vi "PixyGetCube.vi"(10 "AbortButtonPushed":bool, 11 "CubeGrabButtonPushed":bool) -> (3 "GotCube?":bool)   [LabVIEW 2017]
uses:
  <vilib>/Rock Robotics/SystemInterfaces/i2clib/i2c_bus.ctl
panel:
  in  "EndCondArea":i32=11000
  in  "CenterSetpoint":i32=80
  in  "AreaSetpoint":i32
  in  "MaxY":i32=130
  in  "KdX":dbl=0.07
  in  "MaxSpeed":dbl=0.3
  in  "KpX":dbl=0.1
  in  "KpY":dbl=0.0001
  in  "Pixy Address":u8=84 format="%x"
  # "320 x 200"
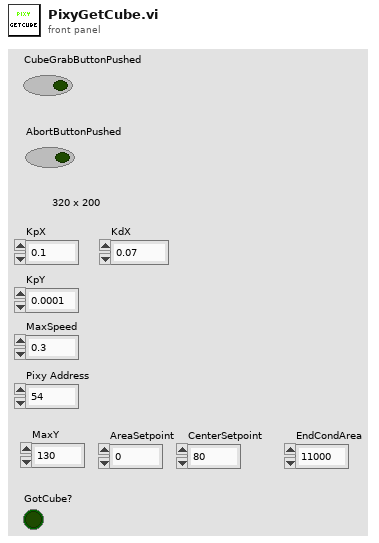
[diagram p1: front panel]
types:
  T1 = typedef "i2c_bus.ctl" = enum16{"I2C On-Board", "I2C MXP", "Invalid"}
  T2 = typedef "WPI_MotorControlDeviceRef.ctl" = cluster{"DeviceStatus":errorcluster, "Type":T3, "PWM":cluster{"PWM Channel":T4, "DeadBand":T5}, "CAN":cluster{"Device Number":u8, "SetOutput VI Ref":variant, "GetOutput VI Ref":variant, "Enable VI Ref":variant, "Disable VI Ref":variant, "Data":variant}, "Invert":bool, "DIO PWM":cluster{"PWM \"Enable\" Channel":T4, "DIOChannel":T6, "PWM Rate":dbl}}
  T3 = typedef "WPI_MotorControlType.ctl" = enum16{"PWM", "CAN", "DIO PWM"}
  T4 = typedef "FPGA_DIOPWMChannel.ctl" = enum8{"PWM 0", "PWM 1", "PWM 2", "PWM 3", "PWM 4", "PWM 5", "PWM 6", "PWM 7", "PWM 8", "PWM 9", "PWM MXP 0", "PWM MXP 1", "PWM MXP 2", "PWM MXP 3", "PWM MXP 4", "PWM MXP 5", "PWM MXP 6", "PWM MXP 7", "PWM MXP 8", "PWM MXP 9", "Invalid"}
  T5 = typedef "WPI_PWMDeadband.ctl" = cluster{"Name":string, "maxPositivePwm":i32, "minPositivePwm":i32, "centerPwm":i32, "maxNegativePwm":i32, "minNegativePwm":i32, "angularRange":u16}
  T6 = typedef "FPGA_DIOChannel.ctl" = enum8{"DIO 0", "DIO 1", "DIO 2", "DIO 3", "DIO 4", "DIO 5", "DIO 6", "DIO 7", "DIO 8", "DIO 9", "DIO MXP 0", "DIO MXP 1", "DIO MXP 2", "DIO MXP 3", "DIO MXP 4", "DIO MXP 5", "DIO MXP 6", "DIO MXP 7", "DIO MXP 8", "DIO MXP 9", "DIO MXP 10", "DIO MXP 11", "DIO MXP 12", "DIO MXP 13", "DIO MXP 14", "DIO MXP 15", "SPI Port CS1", "SPI Port CS2", "SPI Port CS3", "SPI Port MISO", "SPI Port MOSI", "Invalid"}
  T7 = typedef "WPI_I2CDevRef.ctl" = cluster{"DevStatus":errorcluster, "Device Address":u8, "Handle":i32, "I2C Bus":T1}
  T8 = cluster{"MotorControlDevRef":T2, "MotorControlDevRef":T2}
  T9 = cluster{"MotorControlDevRef":T2, "MotorControlDevRef":T2, "MotorControlDevRef":T2, "MotorControlDevRef":T2}
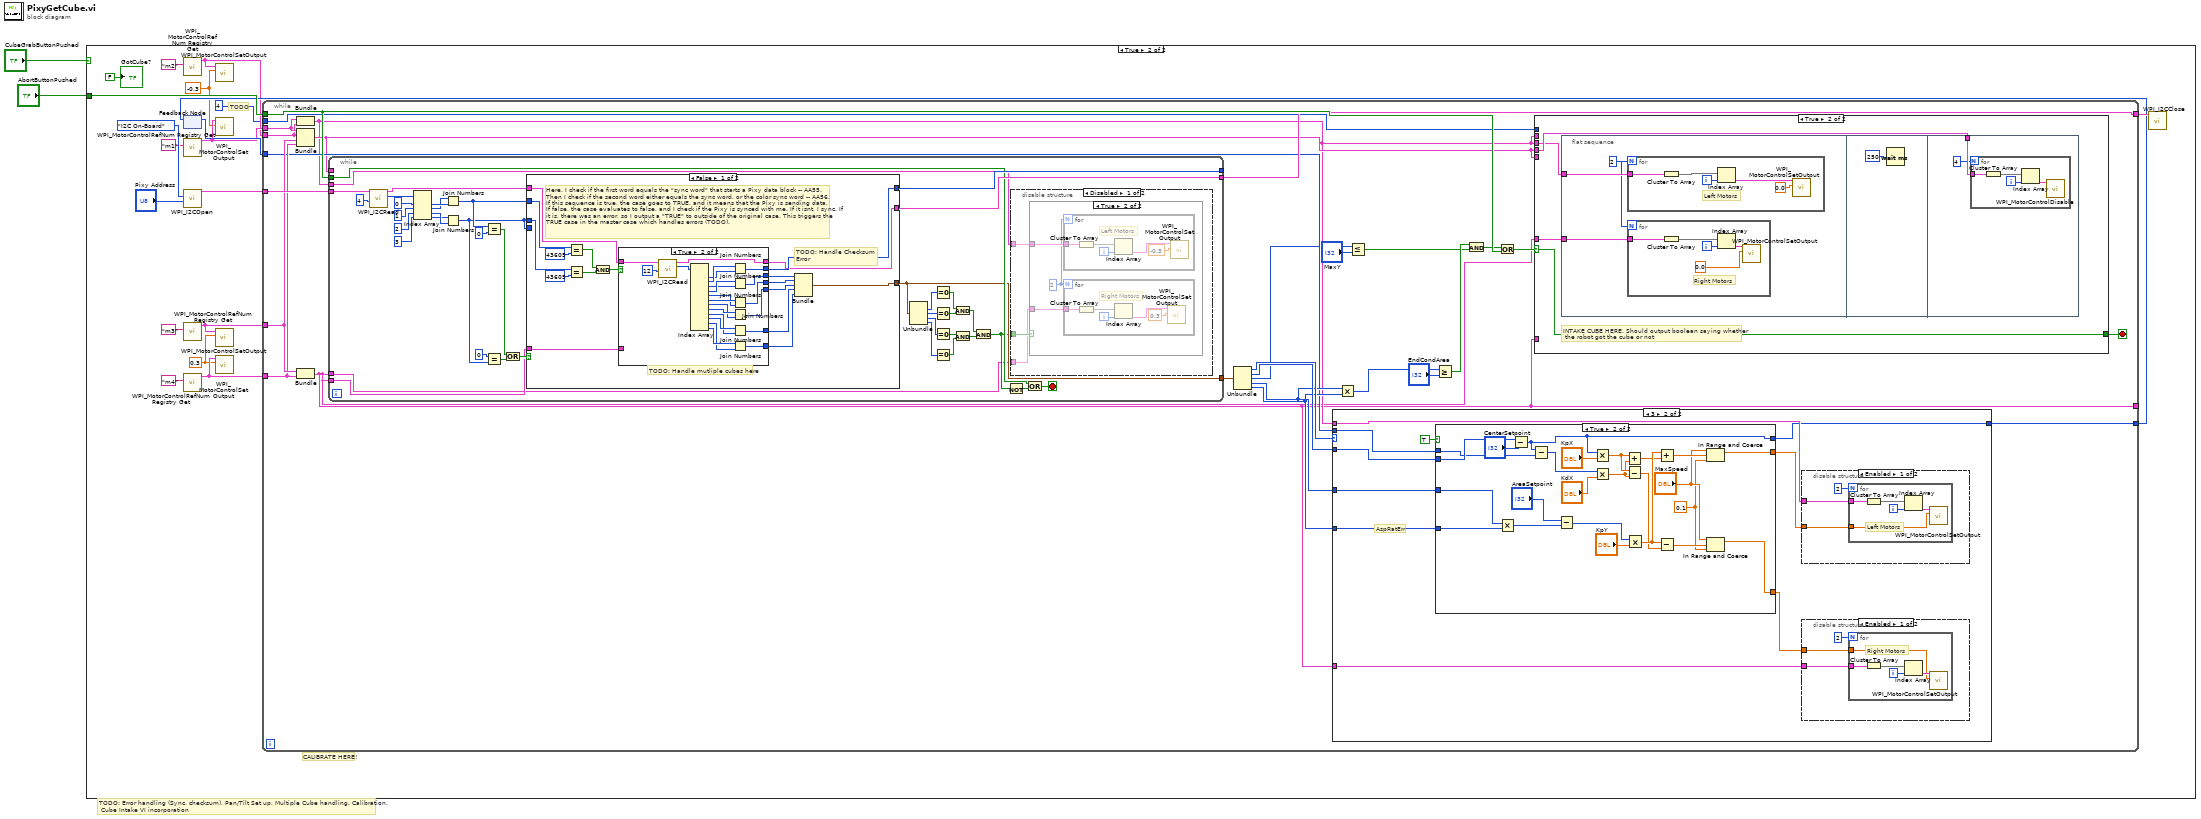
[diagram p0: block diagram]
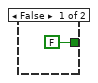
[diagram p3: hidden frame]
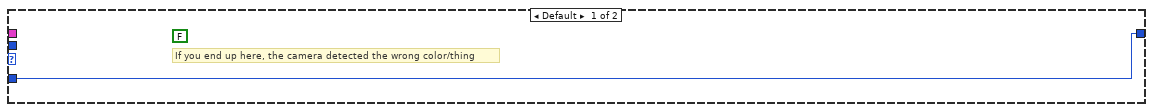
[diagram p4: hidden frame]
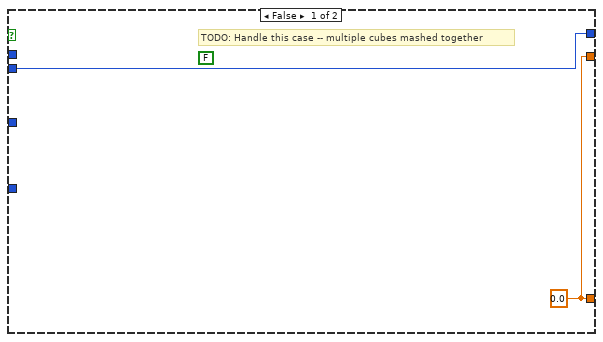
[diagram p7: hidden frame]
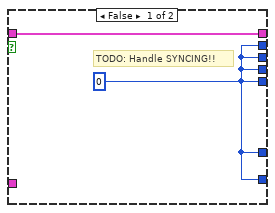
[diagram p10: hidden frame]
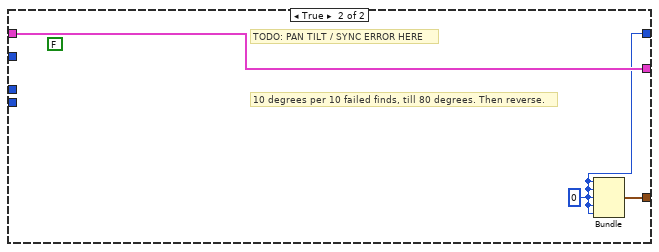
[diagram p11: hidden frame]
diagram:
  # "TODO: Error handling (Sync, checksum), Pan/Tilt Set up, Multiple Cube handling, Calibration,\n Cube Intake VI incorporation"
  n1 = case shown="True" "CubeGrabButtonPushed" {
    tunnel: "AbortButtonPushed" -> [_ w21]
    frame False {
    }
    frame True {
      w4 = -0.3 ("Output")
      w7 = 0.3 ("Output")
      # "TODO"
      # "CALIBRATE HERE!"
      n2 = call <vilib>:"WPI_MotorControlRefNum Registry Get.vi"("refnum name"="m2") -> ("MotorControlDevRef"=w5:T2)  [unwired: 9 in, 1 out]
      n3 = feedback #1() -> (w11:i32)  [unwired: 1 in]
      n4 = call <vilib>:"WPI_MotorControlRefNum Registry Get.vi"("refnum name"="m1") -> ("MotorControlDevRef"=w6:T2)  [unwired: 9 in, 1 out]
      n5 = call <vilib>:"WPI_I2COpen.vi"("Device Address"="Pixy Address", "I2C Bus"=i2c_bus."I2C On-Board") -> ("I2CDevRef"=w12:T7)  [unwired: 8 in, 1 out]
      n6 = call <vilib>:"WPI_MotorControlRefNum Registry Get.vi"("refnum name"="m3") -> ("MotorControlDevRef"=w9:T2)  [unwired: 9 in, 1 out]
      n7 = call <vilib>:"WPI_MotorControlRefNum Registry Get.vi"("refnum name"="m4") -> ("MotorControlDevRef"=w8:T2)  [unwired: 9 in, 1 out]
      n8 = call <vilib>:"WPI_MotorControlSetOutput.vi"("Output"=w4, "MotorControlDevRef"=w5) -> ()  [unwired: 7 in, 3 out]
      n9 = call <vilib>:"WPI_MotorControlSetOutput.vi"("Output"=w4, "MotorControlDevRef"=w6) -> ()  [unwired: 7 in, 3 out]
      n10 = call <vilib>:"WPI_MotorControlSetOutput.vi"("Output"=w7, "MotorControlDevRef"=w9) -> ()  [unwired: 7 in, 3 out]
      n11 = call <vilib>:"WPI_MotorControlSetOutput.vi"("Output"=w7, "MotorControlDevRef"=w8) -> ()  [unwired: 7 in, 3 out]
      n12 = while {
        tunnel: w21 -> [w48]
        tunnel: w5 -> [w39]
        tunnel: w6 -> [w40]
        tunnel: w8 -> [w37]
        tunnel: w9 -> [w38]
        tunnel: [w47] -> w18
        tunnel: w12 -> [w46]
        tunnel: [w24] -> _
        tunnel: w11 -> [w36]
        tunnel: [w35] -> w10
        tunnel: 4 -> [w27]
        stop <- w28 stop-if-true
        n13 = Bundle("MotorControlDevRef"=w40, "MotorControlDevRef"=w39) -> (w25:T8)  [unwired: 1 in]
        n14 = Bundle("MotorControlDevRef"=w40, "MotorControlDevRef"=w39, "MotorControlDevRef"=w38, "MotorControlDevRef"=w37) -> (w26:T9)  [unwired: 1 in]
        n15 = Bundle("MotorControlDevRef"=w38, "MotorControlDevRef"=w37) -> (w24:T8)  [unwired: 1 in]
        n16 = while {
          tunnel: w48 -> [w143]
          tunnel: w46 -> [w151]
          tunnel: [w146] -> _
          tunnel: [w145] -> w47
          tunnel: w24 -> [w144]
          tunnel: [w131] -> w43
          tunnel: w26 -> [_]
          tunnel: w25 -> [w128]
          tunnel: w24 -> [w127]
          stop <- w132 stop-if-true
          n17 = call <vilib>:"WPI_I2CRead.vi"("I2CBytesToRead"=u8 4, "I2CDevRef"=w151) -> ("Data Out"=w160:u8[], "I2CDevRef"=w149:T7)  [unwired: 7 in, 1 out]
          n18 = Index Array(array=w160, index #1=0 ("index"), index #2=1 ("index"), index #3=2 ("index"), index #4=3 ("index")) -> (element #1=w155:u8, element #2=w154:u8, element #3=w153:u8, element #4=w152:u8)
          n19 = Join Numbers(hi=w154, lo=w155) -> ((hi.lo)=w148:u16)
          n20 = Join Numbers(hi=w152, lo=w153) -> ((hi.lo)=w147:u16)
          n21 = Equal?(x=w148, y=u16 0) -> (x = y?=w163:bool)
          n22 = Equal?(x=u16 0, y=w147) -> (x = y?=w162:bool)
          n23 = Or(x=w163, y=w162) -> (x .or. y?=w150:bool)
          n24 = case shown="False" w150 {
            tunnel: w149 -> [w195 w225]
            tunnel: w148 -> [w194 _]
            tunnel: w147 -> [w193 _]
            tunnel: w147 -> [_ _]
            tunnel: [w192 w224] -> w146
            tunnel: [w189 w225] -> w145
            tunnel: [w183 w223] -> w131
            tunnel: w144 -> [w182 _]
            frame False {
              # "TODO: Handle Checksum \nError"
              # "TODO: Handle mutliple cubes here"
              # "Here, I check if the first word equals the \"sync word\" that starts a Pixy data block -- AA55. \nThen I check if the second word either equals the sync word, or the color sync word -- AA56.\nIf this sequence is true, the case goes to TRUE, and it means that the Pixy is sending data.\nIf false, the case evaluates to false, and I check if the Pixy is synced with me. If it isnt, I sync. If\nit is, there was an error, so I output a \"TRUE\" to outside of the original case. This triggers the \nTRUE case in the master case which handles errors (TODO)."
              n25 = Equal?(x=w194, y=u16 43605) -> (x = y?=w198:bool)
              n26 = Equal?(x=w193, y=u16 43605) -> (x = y?=w191:bool)
              n27 = And(x=w198, y=w191) -> (x .and. y?=w190:bool)
              n28 = case shown="True" w190 {
                tunnel: w195 -> [w199 w222]
                tunnel: [w200 w208] -> w184
                tunnel: [w200 w207] -> w185
                tunnel: [w200 w206] -> w186
                tunnel: [w200 w205] -> w187
                tunnel: [w200 w204] -> w188
                tunnel: [w200 w203] -> w192
                tunnel: [w199 w201] -> w189
                tunnel: w182 -> [_ _]
                frame False {
                  w200 = 0
                  # "TODO: Handle SYNCING!!"
                }
                frame True {
                  n29 = call <vilib>:"WPI_I2CRead.vi"("I2CBytesToRead"=u8 12, "I2CDevRef"=w222) -> ("Data Out"=w202:u8[], "I2CDevRef"=w201:T7)  [unwired: 7 in, 1 out]
                  n30 = Index Array(array=w202) -> (element #1=w209:u8, element #2=w210:u8, element #3=w211:u8, element #4=w212:u8, element #5=w213:u8, element #6=w214:u8, element #7=w215:u8, element #8=w216:u8, element #9=w217:u8, element #10=w218:u8, element #11=w219:u8, element #12=w220:u8)  [unwired: 12 in]
                  n31 = Join Numbers(hi=w210, lo=w209) -> ((hi.lo)=w203:u16)
                  n32 = Join Numbers(hi=w212, lo=w211) -> ((hi.lo)=w204:u16)
                  n33 = Join Numbers(hi=w214, lo=w213) -> ((hi.lo)=w205:u16)
                  n34 = Join Numbers(hi=w216, lo=w215) -> ((hi.lo)=w206:u16)
                  n35 = Join Numbers(hi=w218, lo=w217) -> ((hi.lo)=w207:u16)
                  n36 = Join Numbers(hi=w220, lo=w219) -> ((hi.lo)=w208:u16)
                }
              }
              n37 = Bundle(w188, w187, w186, w185, w184) -> (w183:cluster{i32, i32, i32, i32, i32})  [unwired: 1 in]
            }
            frame True {
              (unwired) FALSE
              w224 = 0
              # "10 degrees per 10 failed finds, till 80 degrees. Then reverse."
              # "TODO: PAN TILT / SYNC ERROR HERE"
              n38 = Bundle(w224, w224, w224, w224, w224) -> (w223:cluster{i32, i32, i32, i32, i32})  [unwired: 1 in]
            }
          }
          n39 = Unbundle(w131) -> (w142:i32, w141:i32, w140:i32, w139:i32)  [unwired: 1 out]
          n40 = Equal To 0?(x=w142) -> (x = 0?=w130:bool)
          n41 = Equal To 0?(x=w141) -> (x = 0?=w138:bool)
          n42 = Equal To 0?(x=w140) -> (x = 0?=w137:bool)
          n43 = Equal To 0?(x=w139) -> (x = 0?=w136:bool)
          n44 = And(x=w130, y=w138) -> (x .and. y?=w134:bool)
          n45 = And(x=w137, y=w136) -> (x .and. y?=w133:bool)
          n46 = And(x=w134, y=w133) -> (x .and. y?=w129:bool)
          n47 = Not(x=w129) -> (.not. x?=w135:bool)
          n48 = disable-structure shown="Disabled" {
            disable-tunnel: w129 -> [w168 _]
            disable-tunnel: w128 -> [w167 _]
            disable-tunnel: w127 -> [w166 _]
            frame Disabled {
              n49 = case shown="True" w168 {
                tunnel: w167 -> [_ w171]
                tunnel: w166 -> [_ w170]
                frame False {
                }
                frame True {
                  w169 = 2
                  n50 = for {
                    N: w169 -> [_]
                    tunnel: w171 -> [w178]
                    i -> [w179]
                    # "Left Motors"
                    n51 = Cluster To Array(cluster=w178) -> (array=w181:T2[])
                    n52 = Index Array(array=w181, index=w179) -> (element=w180:T2)
                    n53 = call <vilib>:"WPI_MotorControlSetOutput.vi"("Output"=-0.3, "MotorControlDevRef"=w180) -> ()  [unwired: 7 in, 3 out]
                  }
                  n54 = for {
                    N: w169 -> [_]
                    tunnel: w170 -> [w173]
                    i -> [w174]
                    # "Right Motors"
                    n55 = Cluster To Array(cluster=w173) -> (array=w176:T2[])
                    n56 = Index Array(array=w176, index=w174) -> (element=w175:T2)
                    n57 = call <vilib>:"WPI_MotorControlSetOutput.vi"("Output"=0.3, "MotorControlDevRef"=w175) -> ()  [unwired: 7 in, 3 out]
                  }
                }
              }
            }
            frame Enabled {
            }
          }
          n58 = Or(x=w143, y=w135) -> (x .or. y?=w132:bool)
        }
        n59 = Unbundle(w43) -> (w45:i32, w44:i32, w30:i32, w42:i32, w41:i32)
        n60 = case shown="3" w45 {
          tunnel: w24 -> [_ w84]
          tunnel: w25 -> [_ w83]
          tunnel: w44 -> [w74 w82]
          tunnel: w42 -> [_ w78]
          tunnel: w41 -> [_ w77]
          tunnel: [w74 w76] -> w35
          tunnel: w36 -> [_ w75]
          frame Default {
            (unwired) FALSE
            # "If you end up here, the camera detected the wrong color/thing"
          }
          frame 3 {
            # "AspRatErr"
            n61 = case shown="True" TRUE {
              tunnel: w82 -> [w101 w118]
              tunnel: [w102 w119] -> w80
              tunnel: [w102 w120] -> w81
              tunnel: w78 -> [_ w126]
              tunnel: w77 -> [_ w125]
              tunnel: [w101 w111] -> w76
              tunnel: w75 -> [_ w110]
              frame False {
                (unwired) FALSE
                w102 = 0.0
                # "TODO: Handle this case -- multiple cubes mashed together"
              }
              frame True {
                w105 = 0.1 ("lower limit")
                n62 = Multiply(x=w126, y=w125) -> (x*y=w116:i32)
                n63 = Subtract(x=w118, y="CenterSetpoint") -> (x-y=w111:i32)
                n64 = Subtract(x=w111, y=w110) -> (x-y=w112:i32)
                n65 = Subtract(x="AreaSetpoint", y=w116) -> (x-y=w115:i32)
                n66 = Multiply(x=w111, y="KpX") -> (x*y=w109:dbl)
                n67 = Multiply(x=w112, y="KdX") -> (x*y=w108:dbl)
                n68 = Add(x=w109, y=w108) -> (x+y=w113:dbl)
                n69 = Subtract(x=w109, y=w108) -> (x-y=w107:dbl)
                n70 = Multiply(x=w115, y="KpY") -> (x*y=w117:dbl)
                n71 = Add(x=w117, y=w113) -> (x+y=w122:dbl)
                n72 = Subtract(x=w117, y=w107) -> (x-y=w121:dbl)
                n73 = In Range and Coerce(upper limit="MaxSpeed", x=w122, lower limit=w105) -> (coerced(x)=w119:dbl)  [unwired: 1 out]
                n74 = In Range and Coerce(upper limit="MaxSpeed", x=w121, lower limit=w105) -> (coerced(x)=w120:dbl)  [unwired: 1 out]
              }
            }
            n75 = disable-structure shown="Enabled" {
              disable-tunnel: w83 -> [w94 _]
              disable-tunnel: w80 -> [w93 _]
              frame Enabled {
                n76 = for {
                  N: 2 -> [_]
                  tunnel: w94 -> [w96]
                  tunnel: w93 -> [w97]
                  i -> [w98]
                  # "Left Motors"
                  n77 = Cluster To Array(cluster=w96) -> (array=w100:T2[])
                  n78 = Index Array(array=w100, index=w98) -> (element=w99:T2)
                  n79 = call <vilib>:"WPI_MotorControlSetOutput.vi"("Output"=w97, "MotorControlDevRef"=w99) -> ()  [unwired: 7 in, 3 out]
                }
              }
              frame Disabled {
              }
            }
            n80 = disable-structure shown="Enabled" {
              disable-tunnel: w84 -> [w86 _]
              disable-tunnel: w81 -> [w85 _]
              frame Enabled {
                n81 = for {
                  N: 2 -> [_]
                  tunnel: w86 -> [w88]
                  tunnel: w85 -> [w89]
                  i -> [w91]
                  # "Right Motors"
                  n82 = Cluster To Array(cluster=w88) -> (array=w92:T2[])
                  n83 = Index Array(array=w92, index=w91) -> (element=w90:T2)
                  n84 = call <vilib>:"WPI_MotorControlSetOutput.vi"("Output"=w89, "MotorControlDevRef"=w90) -> ()  [unwired: 7 in, 3 out]
                }
              }
              frame Disabled {
              }
            }
          }
        }
        n85 = Multiply(x=w42, y=w41) -> (x*y=w31:i32)
        n86 = Less Or Equal?(x=w30, y="MaxY") -> (x <= y?=w32:bool)
        n87 = Greater Or Equal?(x=w31, y="EndCondArea") -> (x >= y?=w34:bool)
        n88 = And(x=w34, y=w32) -> (x .and. y?=w33:bool)
        n89 = Or(x=w33, y=w48) -> (x .or. y?=w29:bool)
        n90 = case shown="True" w29 {
          selector: w29 -> [_ w53]
          tunnel: w27 -> [_ _]
          tunnel: w26 -> [_ _]
          tunnel: [FALSE w53] -> w28
          tunnel: w25 -> [_ _]
          tunnel: w24 -> [_ _]
          tunnel: w26 -> [_ w52]
          tunnel: w25 -> [_ w51]
          tunnel: w24 -> [_ w50]
          frame False {
          }
          frame True {
            # "INTAKE CUBE HERE. Should output boolean saying whether\n the robot got the cube or not"
            n91 = flat-sequence {
              tunnel: w51 -> [w56]
              tunnel: w50 -> [w55]
              tunnel: w52 -> [w69]
              frame #0 {
                w54 = 2
                n92 = for {
                  N: w54 -> [_]
                  tunnel: w56 -> [w63]
                  i -> [w64]
                  # "Left Motors"
                  n93 = Cluster To Array(cluster=w63) -> (array=w66:T2[])
                  n94 = Index Array(array=w66, index=w64) -> (element=w65:T2)
                  n95 = call <vilib>:"WPI_MotorControlSetOutput.vi"("Output"=0.0, "MotorControlDevRef"=w65) -> ()  [unwired: 7 in, 3 out]
                }
                n96 = for {
                  N: w54 -> [_]
                  tunnel: w55 -> [w58]
                  i -> [w60]
                  # "Right Motors"
                  n97 = Cluster To Array(cluster=w58) -> (array=w61:T2[])
                  n98 = Index Array(array=w61, index=w60) -> (element=w59:T2)
                  n99 = call <vilib>:"WPI_MotorControlSetOutput.vi"("Output"=0.0, "MotorControlDevRef"=w59) -> ()  [unwired: 7 in, 3 out]
                }
              }
              frame #1 {
                n100 = Wait (ms)(milliseconds to wait=u32 250) -> ()  [unwired: 1 out]
              }
              frame #2 {
                n101 = for {
                  N: 4 -> [_]
                  tunnel: w69 -> [w71]
                  i -> [w73]
                  n102 = Cluster To Array(cluster=w71) -> (array=w72:T2[])
                  n103 = Index Array(array=w72, index=w73) -> (element=w70:T2)
                  n104 = call <vilib>:"WPI_MotorControlDisable.vi"("MotorControlDevRef"=w70) -> ()  [unwired: 9 in, 2 out]
                }
              }
            }
          }
        }
      }
      n105 = feedback-in #1(w10) -> ()
      n106 = call <vilib>:"WPI_I2CClose.vi"("I2CDevRef"=w18) -> ()  [unwired: 10 in, 1 out]
      "GotCube?" <- FALSE ("GotCube?")
    }
  }
